vi "Toggle UI.vi"(8 "Error in (no error)":errorcluster, 9 "Enabled? (T)":bool=TRUE, 10 "SSID Values Refnum":refnum<vi>, 11 "Submit Button Refnum":refnum<vi>) -> (0 "Error Out":errorcluster)   [LabVIEW 2024]
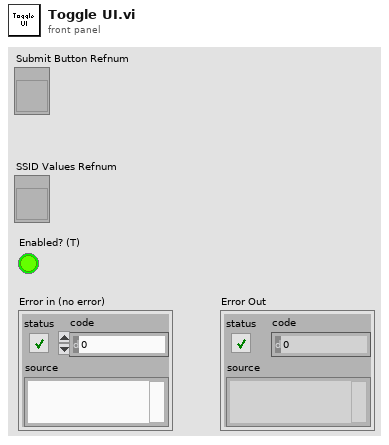
[diagram p1: front panel]
types:
  T1 = enum8{"Enabled", "Disabled", "Disabled and Grayed Out"}
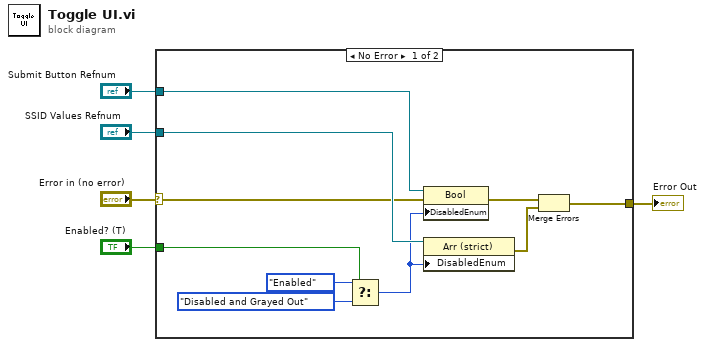
[diagram p0: block diagram]
diagram:
  n1 = case shown="No Error" "Error in (no error)" {
    selector: "Error in (no error)" -> [w8 w16]
    tunnel: "Enabled? (T)" -> [w11 _]
    tunnel: "Submit Button Refnum" -> [w10 _]
    tunnel: "SSID Values Refnum" -> [w9 _]
    tunnel: [w6 w16] -> w1
    frame No Error {
      n2 = Select(t=T1."Enabled", s=w11, f=T1."Disabled and Grayed Out") -> (s? t:f=w7:T1)
      n3 = property on="Property Node" class="Bool"(reference=w10, error in=w8, "DisabledEnum"=w7) -> (error out=w15:errorcluster)  [unwired: 1 out]
      n4 = property on="Property Node" class="Arr (strict)"(reference=w9, "DisabledEnum"=w7) -> (error out=w14:errorcluster)  [unwired: 1 in, 1 out]
      n5 = Merge Errors(w15, w14) -> (w6:errorcluster)
    }
    frame Error {
    }
  }
  "Error Out" <- w1
